vi "check shift.vi"() -> (3 "Shift":string)   [LabVIEW 2015]
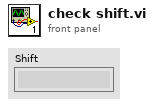
[diagram p1: front panel]
types:
  T1 = cluster{"second":i32, "minute":i32, "hour":i32, "day of month":i32, "month":i32, "year":i32, "day of week":i32, "day of year":i32, "is DST":i32}
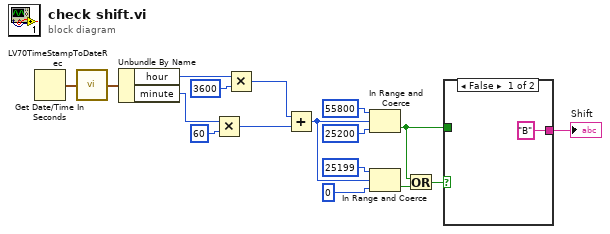
[diagram p0: block diagram]
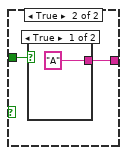
[diagram p2: hidden frame]
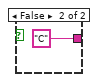
[diagram p3: hidden frame]
diagram:
  n1 = Get Date/Time In Seconds() -> (seconds since 1Jan1904=w5:timestamp)
  n2 = call <vilib>:"LV70TimeStampToDateRec.vi"("time stamp"=w5) -> ("date time rec"=w4:T1)
  n3 = Unbundle By Name(w4) -> ("hour"=w3:i32, "minute"=w2:i32)
  n4 = Multiply(x=w2, y=60) -> (x*y=w12:i32)
  n5 = Multiply(x=w3, y=3600) -> (x*y=w13:i32)
  n6 = Add(x=w13, y=w12) -> (x+y=w11:i32)
  n7 = In Range and Coerce(upper limit=55800, x=w11, lower limit=25200) -> (In Range?=w6:bool)  [unwired: 1 out]
  n8 = In Range and Coerce(upper limit=25199, x=w11, lower limit=0 ("upper limit")) -> (In Range?=w15:bool)  [unwired: 1 out]
  n9 = Or(x=w6, y=w15) -> (x .or. y?=w14:bool)
  n10 = case shown="False" w14 {
    tunnel: ["B" w20] -> w1
    tunnel: w6 -> [_ w19]
    frame False {
    }
    frame True {
      n11 = case shown="True" w19 {
        tunnel: ["A" "C"] -> w20
        frame True {
        }
        frame False {
        }
      }
    }
  }
  "Shift" <- w1
